vi "Open Camera By Name.vi"(8 "error in":errorcluster, 10 "Camera":T1, 11 "Gantry in":refnum<class "Gantry Class.lvclass">) -> (0 "error out":errorcluster, 3 "Gantry out":refnum<class "Gantry Class.lvclass">)   [LabVIEW 2011, in "Gantry Class.lvclass"]
uses:
  Gantry Class.lvclass
  Config Manager Class/Type Definitions/Camera Enum.ctl
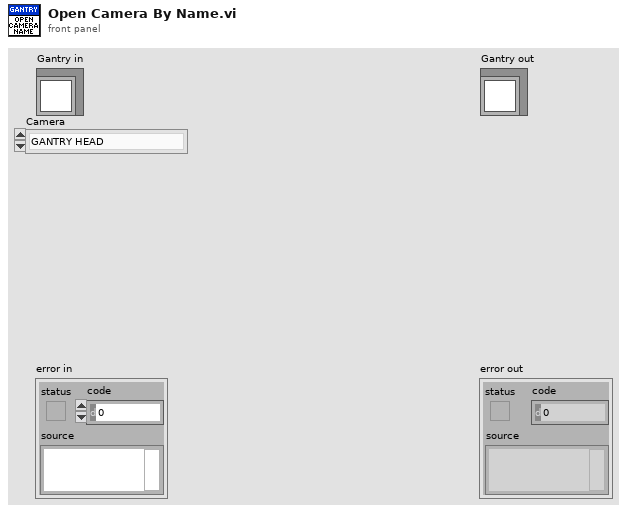
[diagram p1: front panel]
types:
  T1 = typedef "Camera Enum.ctl" = enum16{"GANTRY HEAD", "NEEDLE CALIBRATION X", "NEEDLE CALIBRATION Y"}
  T2 = typedef "Gantry_Camera.ctl" = cluster{"IMAQ Session":T3, "Group":u32, "Open?":bool, "Interface Name":string, "Field of View":cluster{"x-mm":dbl, "y-mm":dbl}, "Name":T1}
  T3 = typedef "IMAQdx.ctl" = refnum<k21>
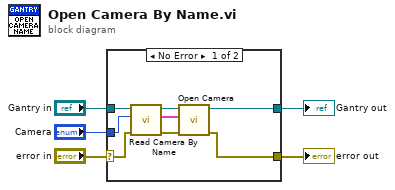
[diagram p0: block diagram]
diagram:
  n1 = case shown="No Error" "error in" {
    selector: "error in" -> [w7 w15]
    tunnel: [w6 w15] -> w4
    tunnel: [w8 w14] -> w2
    tunnel: "Gantry in" -> [w12 w14]
    tunnel: "Camera" -> [w13 _]
    frame No Error {
      n2 = call-dynamic "Read Camera By Name.vi"("error in"=w7, "Camera Name"=w13, "Gantry in"=w12) -> ("error out"=w9:errorcluster, "Camera"=w11:T2, "Gantry out"=w10:refnum<class "Gantry Class.lvclass">)  [unwired: 6 in]
      n3 = call-dynamic "Open Camera.vi"("error in"=w9, "Camera"=w11, "Gantry in"=w10) -> ("error out"=w6:errorcluster, "Gantry out"=w8:refnum<class "Gantry Class.lvclass">)  [unwired: 6 in, 1 out]
    }
    frame Error {
    }
  }
  "error out" <- w4
  "Gantry out" <- w2
